vi "Save_Single_Images_fr_iSpy.vi"(2 "Image name":string="test", 3 "Image directory path":path=path "C:/test", 4 "Camera":string="EnFlo_Trav1") -> (0 "Error out":errorcluster, 1 "Image Path":path)   [LabVIEW 2018]
uses:
  Anemometry/Anemometry Sub Vis/Globals/Constants_global.vi
  Anemometry/Anemometry Sub Vis/Globals/Trav_pos_global.vi
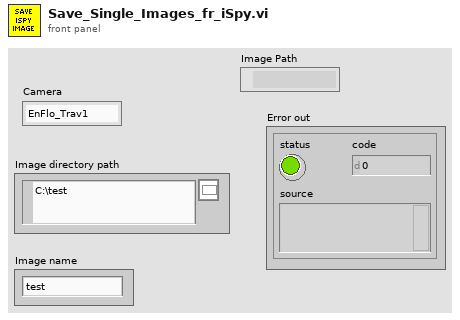
[diagram p1: front panel]
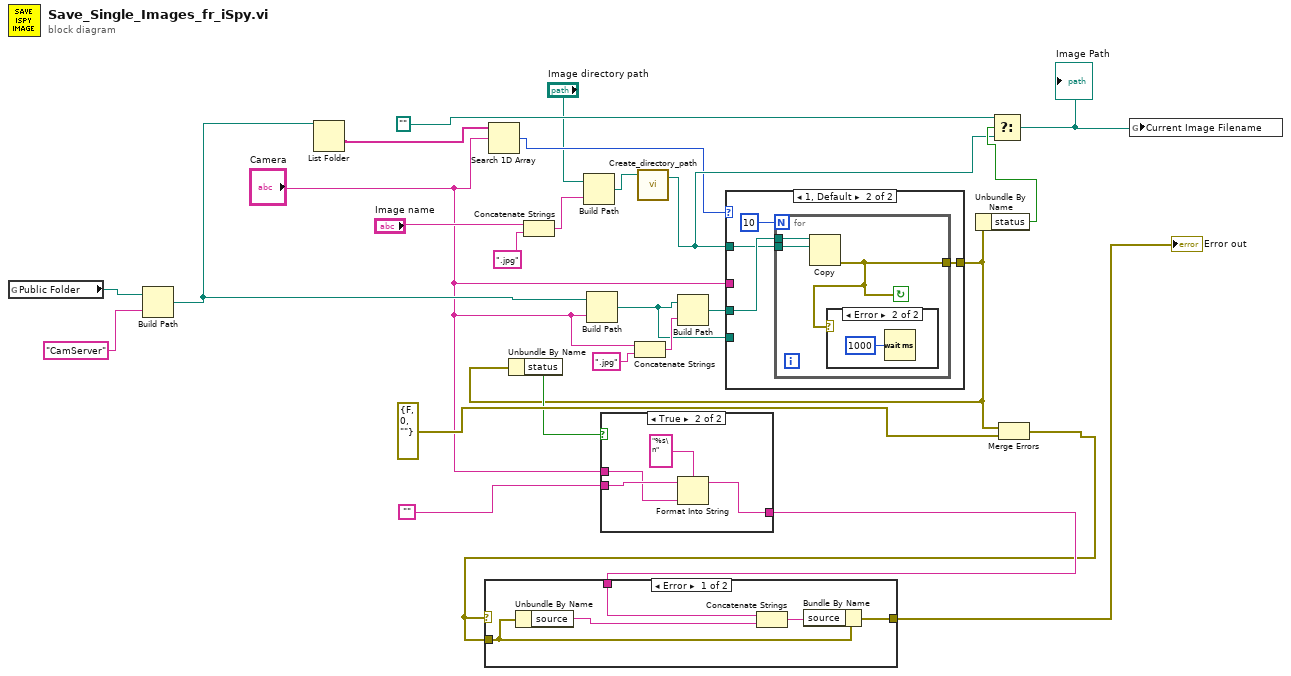
[diagram p0: block diagram]
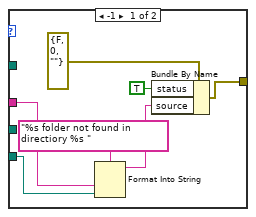
[diagram p2: hidden frame]
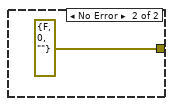
[diagram p5: hidden frame]
diagram:
  n1 = global read "Constants_global.vi" "Public Folder"() -> (w18:path)
  n2 = Build Path(base path=w18, name or relative path="CamServer") -> (appended path=w16:path)
  n3 = List Folder(path=w16) -> (folder names=w17:string[])  [unwired: 3 in, 3 out]
  n4 = Search 1D Array(1D array=w17, element="Camera") -> (index of element=w5:i32)  [unwired: 1 in]
  n5 = Concatenate Strings("Image name", ".jpg" ("string")) -> (w12:string)
  n6 = Build Path(base path="Image directory path", name or relative path=w12) -> (appended path=w11:path)
  n7 = Build Path(base path=w16, name or relative path="Camera") -> (appended path=w4:path)
  n8 = Concatenate Strings("Camera", ".jpg" ("string")) -> (w9:string)
  n9 = call "Create_directory_path.vi"("Path name"=w11) -> ("Path name Out"=w6:path)  [unwired: 2 in, 1 out]
  n10 = Build Path(base path=w4, name or relative path=w9) -> (appended path=w8:path)
  n11 = case shown="1, Default" w5 {
    tunnel: w8 -> [_ w37]
    tunnel: [w32 w36] -> w7
    tunnel: w6 -> [_ w35]
    tunnel: "Camera" -> [w30 _]
    tunnel: w4 -> [w27 _]
    frame -1 {
      n12 = Format Into String(format string="%s folder not found in directiory %s ", w30, w27) -> (resulting string=w29:string)  [unwired: 2 in, 1 out]
      n13 = Bundle By Name(cluster=errorcluster {"status"=FALSE, "code"=0, "source"=""} ("error out"), "status"=TRUE, "source"=w29) -> (w32:errorcluster)
    }
    frame 1, Default {
      n14 = for {
        N: 10 -> [_]
        tunnel: w37 -> [w40]
        tunnel: [w38] -> w36
        tunnel: w35 -> [w39]
        stop <- w38 continue-if-true
        n15 = Copy(10:w39, 11:w40) -> (0:w38:errorcluster)  [unwired: 3 in, 2 out]
        n16 = case shown="Error" w38 {
          frame No Error {
          }
          frame Error {
            n17 = Wait (ms)(milliseconds to wait=u32 1000) -> ()  [unwired: 1 out]
          }
        }
      }
    }
  }
  n18 = Unbundle By Name(w7) -> ("status"=w15:bool)
  n19 = case shown="True" w15 {
    tunnel: [w42 w44] -> w24
    tunnel: "" -> [w42 w46]
    tunnel: "Camera" -> [_ w45]
    frame False {
    }
    frame True {
      n20 = Format Into String(format string="%s\n", initial string=w46, w45) -> (resulting string=w44:string)  [unwired: 1 in, 1 out]
    }
  }
  n21 = Unbundle By Name(w7) -> ("status"=w14:bool)
  n22 = Select(t=path "", s=w14, f=w6) -> (s? t:f=w22:path)
  "Image Path" <- w22
  n23 = Merge Errors(w7, errorcluster {"status"=FALSE, "code"=0, "source"=""} ("error IO")) -> (w20:errorcluster)
  n24 = case shown="Error" w20 {
    tunnel: [w50 errorcluster {"status"=FALSE, "code"=0, "source"=""} ("Error out")] -> w26
    tunnel: w24 -> [w49 _]
    tunnel: w20 -> [w51 _]
    frame Error {
      n25 = Unbundle By Name(w51) -> ("source"=w48:string)
      n26 = Concatenate Strings(w49, w48) -> (w47:string)
      n27 = Bundle By Name(cluster=w51, "source"=w47) -> (w50:errorcluster)
    }
    frame No Error {
    }
  }
  "Error out" <- w26
  n28 = global write "Trav_pos_global.vi" "Current Image Filename"(w22) -> ()
